vi "assemble_command.vi"(5 "stop byte":string, 7 "start byte":string, 9 "data":string, 10 "command code":T1(ring), 11 "operation":enum16{"read", "write", "action"}(ring)) -> (1 "assembled command":string, 2 "checksum":u16, 3 "length":u8, 4 "size of answer":u8, 6 "requires an answer?":bool)   [LabVIEW 2019]
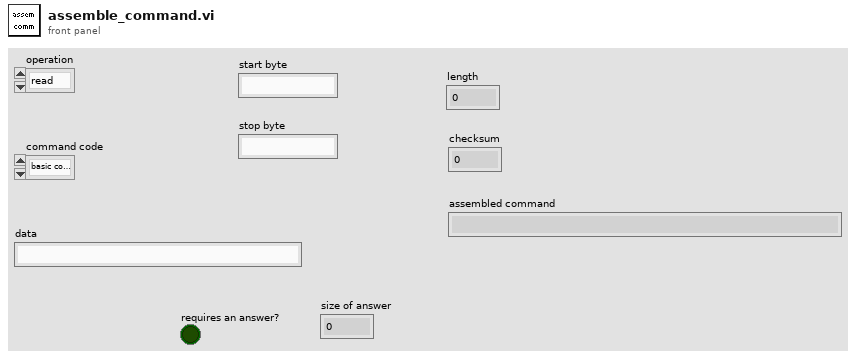
[diagram p1: front panel]
types:
  T1 = enum16{"basic configuration", "test configuration", "converter configuration", "reset", "start", "next cell", "next state"}
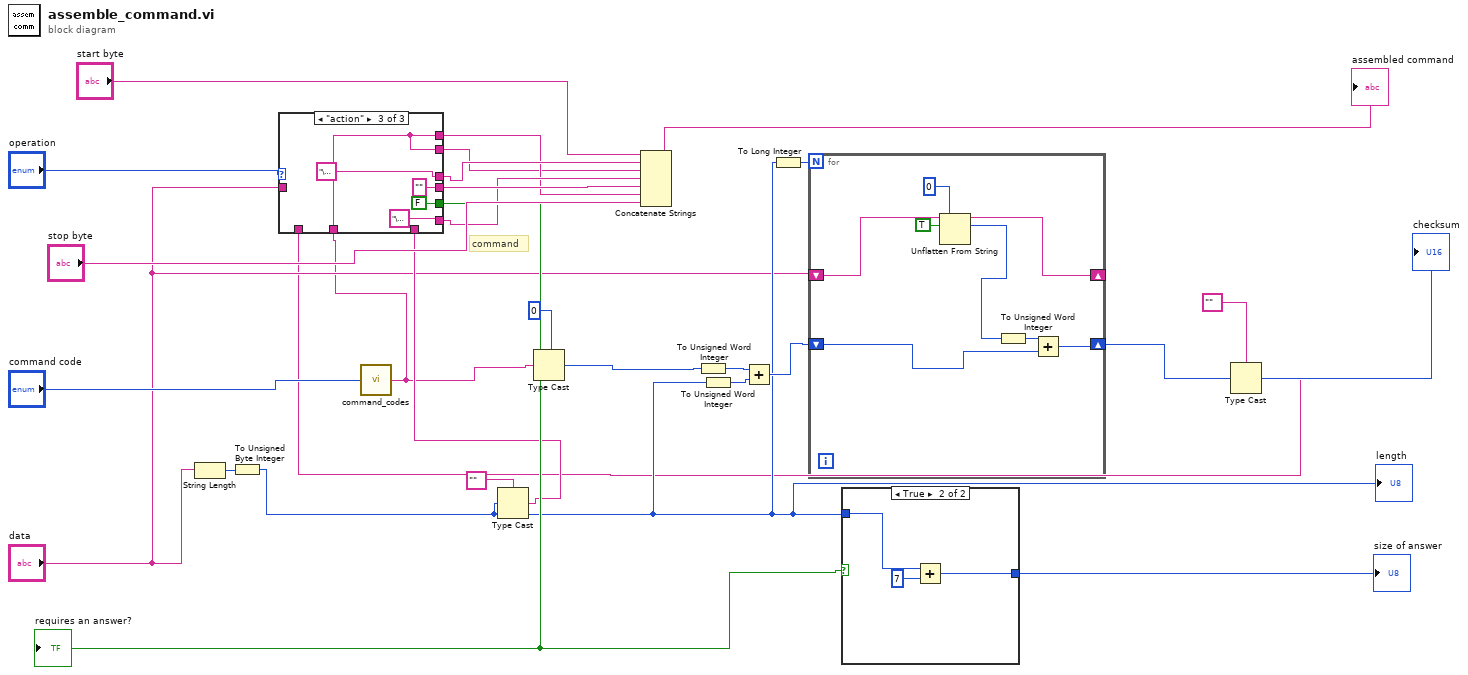
[diagram p0: block diagram]
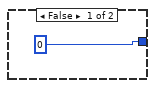
[diagram p2: hidden frame]
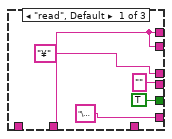
[diagram p3: hidden frame]
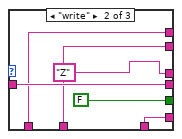
[diagram p4: hidden frame]
diagram:
  # "command"
  n1 = String Length(string="data") -> (length=w10:i32)
  n2 = To Unsigned Byte Integer(number=w10) -> (unsigned 8bit integer=w8:u8)
  "length" <- w8
  n3 = call "command_codes.vi"("command code enum"="command code") -> ("command code"=w2:string)
  n4 = Type Cast(type="", x=w8) -> (*(type *) &x=w6:string)
  n5 = Type Cast(type=u8 0, x=w2) -> (*(type *) &x=w21:u8)
  n6 = To Unsigned Word Integer(number=w21) -> (unsigned 16bit integer=w22:u16)
  n7 = To Unsigned Word Integer(number=w8) -> (unsigned 16bit integer=w23:u16)
  n8 = Add(x=w22, y=w23) -> (x+y=w19:u16)
  n9 = To Long Integer(number=w8) -> (32bit integer=w18:i32)
  n10 = for {
    N: w18 -> [_]
    shift-right: [w30] -> w26
    shift-left: w19 -> [w35]
    shift-right: [w31] -> _
    shift-left: "data" -> [w34]
    n11 = Unflatten From String(type=u8 0, binary string=w34, data includes array or string size? (T)=TRUE) -> (rest of the binary string=w31:string, value=w28:u8)  [unwired: 2 in, 1 out]
    n12 = To Unsigned Word Integer(number=w28) -> (unsigned 16bit integer=w29:u16)
    n13 = Add(x=w29, y=w35) -> (x+y=w30:u16)
  }
  "checksum" <- w26
  n14 = Type Cast(type="", x=w26) -> (*(type *) &x=w3:string)
  n15 = case shown="\"action\"" "operation" {
    tunnel: ["¥" "Z" "\u000f"] -> w15
    tunnel: [TRUE FALSE FALSE] -> w12
    tunnel: "data" -> [_ w44 _]
    tunnel: ["" ("data") w44 "" ("data")] -> w9
    tunnel: ["\u0000" ("data") w43 "\u0000" ("type")] -> w7
    tunnel: w6 -> [_ w43 _]
    tunnel: [w36 w41 w47] -> w4
    tunnel: w3 -> [_ w41 _]
    tunnel: w2 -> [w36 w42 w47]
    tunnel: [w36 w42 w47] -> w1
    frame "read", Default {
    }
    frame "write" {
    }
    frame "action" {
    }
  }
  "requires an answer?" <- w12
  n16 = Concatenate Strings("start byte", w15, w1, w7, w9, w4, "stop byte") -> (→"assembled command":string)
  n17 = case shown="True" w12 {
    tunnel: [u8 0 w54] -> w13
    tunnel: w8 -> [_ w53]
    frame False {
    }
    frame True {
      n18 = Add(x=w53, y=u8 7) -> (x+y=w54:u8)
    }
  }
  "size of answer" <- w13
